vi "Stop Core.vi"(10 "final error code":i32, 11 "Communication Clients in":refnum<class "Communication Clients.lvclass">) -> (3 "Communication Clients out":refnum<class "Communication Clients.lvclass">)   [LabVIEW 2017, in "Communication Clients.lvlib" / "Communication Clients.lvclass"]
doc: "(<B>Filename</B>: Actor Framework.lvlib:Actor.lvclass:Stop Core.vi)\n\nDefines what the actor does before it stops. Use the <B>final error code</B> input to determine whether the actor shut down in response to an error.\n\nBy default, this method does nothing. A descendant class may override it to define behavior, such as shutting down any processes the actor initiated in its override of the Actor Core method."
uses:
  Communication Clients.lvclass
  Communication Clients.lvclass/Communication Clients.ctl
  <vilib>/ActorFramework/Message Enqueuer/Message Enqueuer.lvclass/Message Enqueuer.ctl
  <vilib>/ActorFramework/Message Enqueuer/Enqueue.vi
  <vilib>/ActorFramework/Stop Msg/Stop Msg.lvclass
  C:/Program Files (x86)/National Instruments/LabVIEW 2017/vi.lib/ActorFramework/Message/Message.lvclass
  <vilib>/ActorFramework/Message Priority Queue/Priority Enqueue.vi
  <vilib>/ActorFramework/Actor/Actor.lvclass
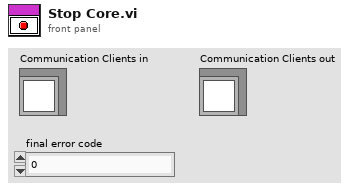
[diagram p1: front panel]
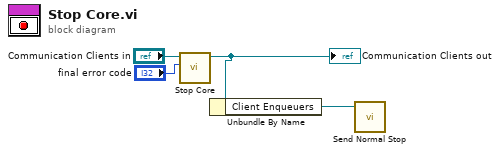
[diagram p0: block diagram]
diagram:
  n1 = call-parent "Stop Core.vi"("final error code"="final error code", "Actor in"="Communication Clients in") -> ("Actor out"=w2:refnum<class "Communication Clients.lvclass">)  [unwired: 9 in]
  "Communication Clients out" <- w2
  n2 = Unbundle By Name(w2) -> ("Client Enqueuers"=w1:refnum<class "Message Enqueuer.lvclass">)
  n3 = call <vilib>:"Send Normal Stop.vi"("Message Enqueuer"=w1) -> ()  [unwired: 10 in, 1 out]
